vi "Read Threshold.vi"(8 "error in (no error)":errorcluster, 11 "Kalman_Filter in":refnum<class "Kalman_Filter.lvclass">) -> (0 "error out":errorcluster, 2 "Threshold":dbl, 3 "Kalman_Filter out":refnum<class "Kalman_Filter.lvclass">)   [LabVIEW 2021, in "Kalman_Filter.lvclass"]
uses:
  Kalman_Filter.lvclass
  Kalman_Filter.lvclass/Kalman_Filter.ctl
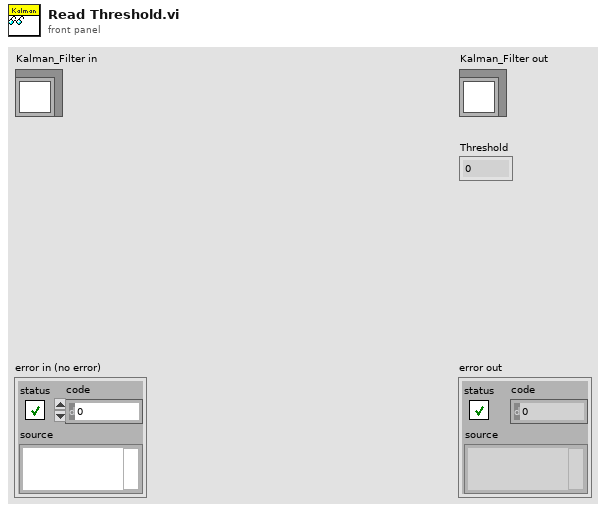
[diagram p1: front panel]
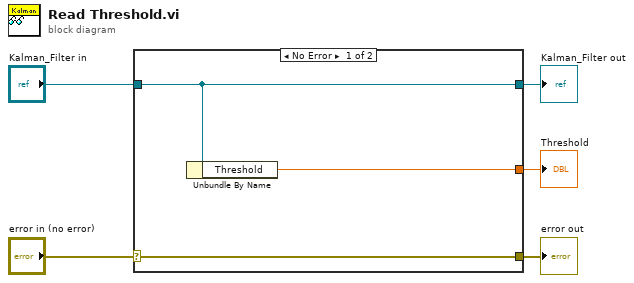
[diagram p0: block diagram]
diagram:
  n1 = case shown="No Error" "error in (no error)" {
    selector: "error in (no error)" -> [w8 w9]
    tunnel: [w8 w9] -> w4
    tunnel: [w7 w10] -> w2
    tunnel: "Kalman_Filter in" -> [w7 w10]
    tunnel: [w6 _] -> w1
    frame No Error {
      n2 = Unbundle By Name(w7) -> ("Threshold"=w6:dbl)
    }
    frame Error {
    }
  }
  "error out" <- w4
  "Kalman_Filter out" <- w2
  "Threshold" <- w1
